vi "Handle Error.vi"(8 "error in (no error)":errorcluster, 11 "DAQMan in":refnum<class "Cfg Grandmaster.lvclass">) -> (0 "error out":errorcluster, 2 "stop actor?":bool=TRUE, 3 "DAQMan out":refnum<class "Cfg Grandmaster.lvclass">)   [LabVIEW 2012, in "Configuration Grandmaster.lvlib" / "Cfg Grandmaster.lvclass"]
doc: "(<B>Filename</B>: Actor Framework.lvlib:Actor.lvclass:Handle Error.vi)\n\nDefines how the actor handles an error that occurred while processing a message.\n\nBy default, this method does nothing except stop the actor. This method also treats error code 43 (coming from <B>error in</B>) as a sign that the actor shut down normally. In this situation, the Handle Error method does not return the error on <B>error out</B>, meaning the actor's caller will not receive it. All other error codes will be returned on <B>error out</B>.\n\nA descendant class may override this method to change this behavior."
uses:
  Cfg Grandmaster.lvclass
  Cfg Grandmaster.lvclass/Cfg Grandmaster.ctl
  Actor Nest/Class Actor Nest/Actor Nest.lvclass
  Class FP Ctrls/FP Controls.lvclass
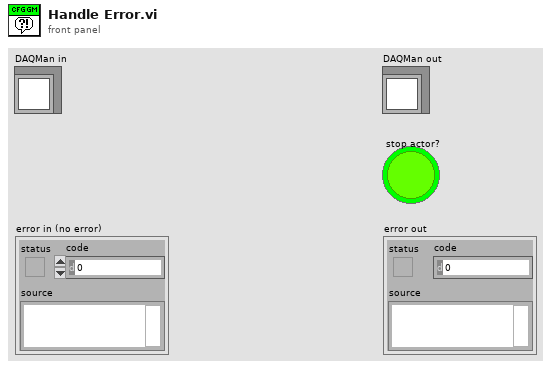
[diagram p1: front panel]
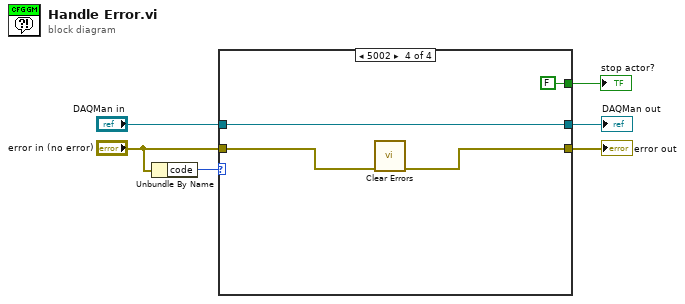
[diagram p0: block diagram]
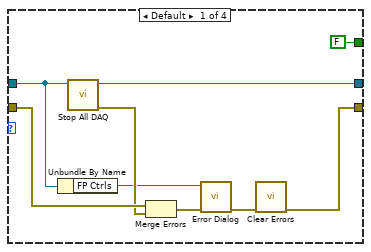
[diagram p2: hidden frame]
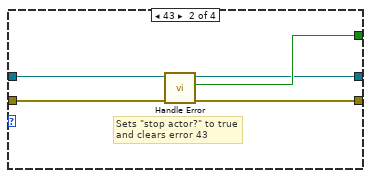
[diagram p3: hidden frame]
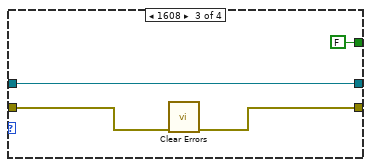
[diagram p4: hidden frame]
diagram:
  n1 = Unbundle By Name("error in (no error)") -> ("code"=w1:i32)
  n2 = case shown="5002" w1 {
    tunnel: [w13 w20 w21 w25] -> w6
    tunnel: [FALSE ("stop actor?") w19 FALSE ("stop actor?") FALSE ("stop actor?")] -> w5
    tunnel: [w14 w18 w23 w27] -> w4
    tunnel: "error in (no error)" -> [w12 w17 w22 w26]
    tunnel: "DAQMan in" -> [w8 w16 w23 w27]
    frame Default {
      n3 = Unbundle By Name(w8) -> ("FP Ctrls"=w7:refnum<class "FP Controls.lvclass">)
      n4 = call "Stop All DAQ.vi"("Cfg Grandmaster in"=w8) -> ("error out"=w11:errorcluster, "Cfg Grandmaster out"=w14:refnum<class "Cfg Grandmaster.lvclass">)  [unwired: 9 in]
      n5 = Merge Errors(w12, w11) -> (w10:errorcluster)
      n6 = call "Error Dialog.vi"("error in"=w10, "FP Controls"=w7) -> ("error out"=w9:errorcluster)  [unwired: 9 in]
      n7 = call <vilib>:"Clear Errors.vi"("error in (no error)"=w9) -> ("error out"=w13:errorcluster)  [unwired: 6 in]
    }
    frame 43 {
      # "Sets \"stop actor?\" to true \nand clears error 43"
      n8 = call-parent "Handle Error.vi"("error in (no error)"=w17, "Actor in"=w16) -> ("error out"=w20:errorcluster, "stop actor?"=w19:bool, "Actor out"=w18:refnum<class "Cfg Grandmaster.lvclass">)  [unwired: 7 in]
    }
    frame 1608 {
      n9 = call <vilib>:"Clear Errors.vi"("error in (no error)"=w22) -> ("error out"=w21:errorcluster)  [unwired: 6 in]
    }
    frame 5002 {
      n10 = call <vilib>:"Clear Errors.vi"("error in (no error)"=w26) -> ("error out"=w25:errorcluster)  [unwired: 6 in]
    }
  }
  "DAQMan out" <- w4
  "error out" <- w6
  "stop actor?" <- w5
